vi "GetAWGStatus.vi"(0 "VISA resource name":refnum<visa-resource-name>, 1 "error in (no error)":errorcluster) -> (2 "VISA resource name out":refnum<visa-resource-name>, 3 "Running":bool, 4 "Waiting For Trigger":bool, 5 "error out":errorcluster)   [LabVIEW 2020, in "Active Technologies AWG3000.lvlib"]
uses:
  Active Technologies AWG3000.lvlib
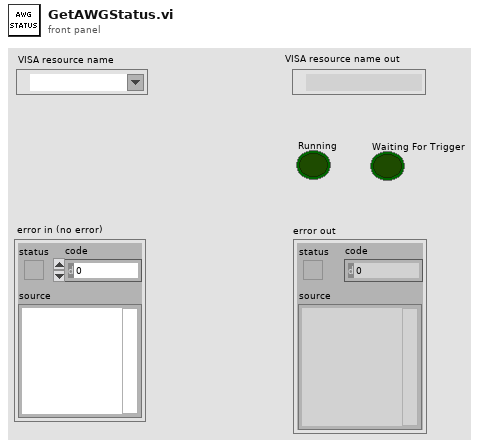
[diagram p1: front panel]
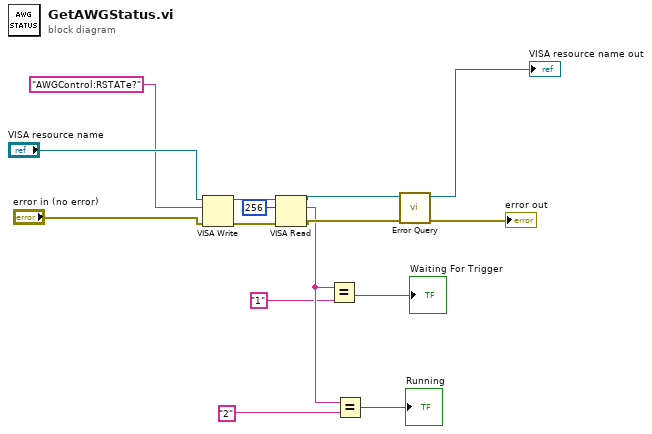
[diagram p0: block diagram]
diagram:
  n1 = VISA Write(VISA resource name="VISA resource name", write buffer="AWGControl:RSTATe?" ("format string"), error in (no error)="error in (no error)") -> (VISA resource name out=w13:refnum<visa-resource-name>, error out=w12:errorcluster)  [unwired: 1 out]
  n2 = VISA Read(VISA resource name=w13, byte count=u32 256, error in (no error)=w12) -> (VISA resource name out=w7:refnum<visa-resource-name>, read buffer=w5:string, error out=w6:errorcluster)  [unwired: 1 out]
  n3 = Equal?(x=w5, y="1") -> (x = y?=→"Waiting For Trigger":bool)
  n4 = Equal?(x=w5, y="2") -> (x = y?=→"Running":bool)
  n5 = call "Error Query.vi"("error in (no error)"=w6, "VISA resource name"=w7) -> ("error out"=→"error out":errorcluster, "VISA resource name out"=→"VISA resource name out":refnum<visa-resource-name>)  [unwired: 6 in, 2 out]
